vi "Splashscreen.vi"(1 "Mode":enum16{"splash", "dialog"}(ring)) -> ()   [LabVIEW 2009]
panel:
  in  "OK Button":bool
  # "PCI"
  # "Physikalisch-Chemisches Institut\nUniversität Heidelberg\nIm Neuenheimer Feld 253"
  # "This software has been developed as tool for optical single molecule spectroscopy within\nthe group of Prof. Dr. J. Wolfrum and Prof. Dr. M. Sauer. It contains all state of the art\ndata acqusition and analysis algorythms developed and used by our workgroup for our \nsingle molecule studies.\n\nThe people mainly involved in these developments through\ndiscussion, experiments and software development are:\n\nDirk-Peter Herten, Philip Tinnefeld, Kenneth D. Weston, Christian Müller,\nChristian Roth, Oliver Piestert and Markus Sauer\n\nPicoQuant HydraHarp modifications by Christian Steinhauer\n\nCopyright (c) 1999, 2000, 2001, 2002, 2003 Physikalisch-Chemisches Institut\nAll rights reserved."
  # "NO WARRANITIES. NOT FOR RESALE.\nCOPIES AND DISTRIBUTION OF THIS SOFTWARE\nIS ONLY ALLOWED WITH EXPLICIT\nPERMITION BY ONE OF ABOVE LISTED PERSONS."
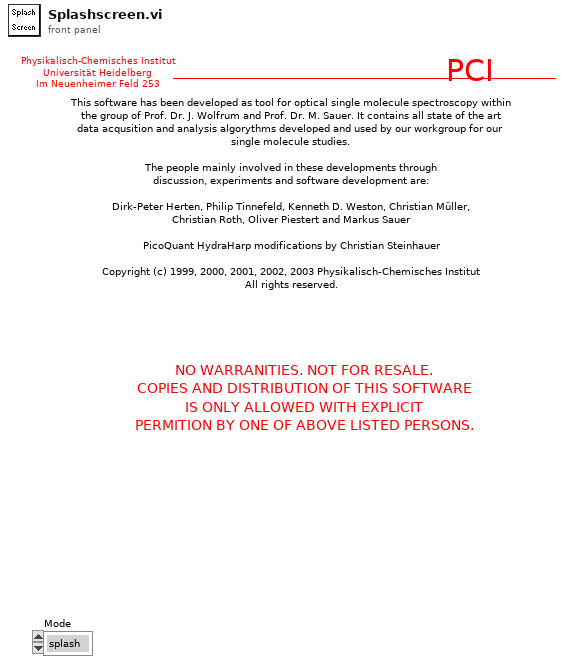
[diagram p1: front panel]
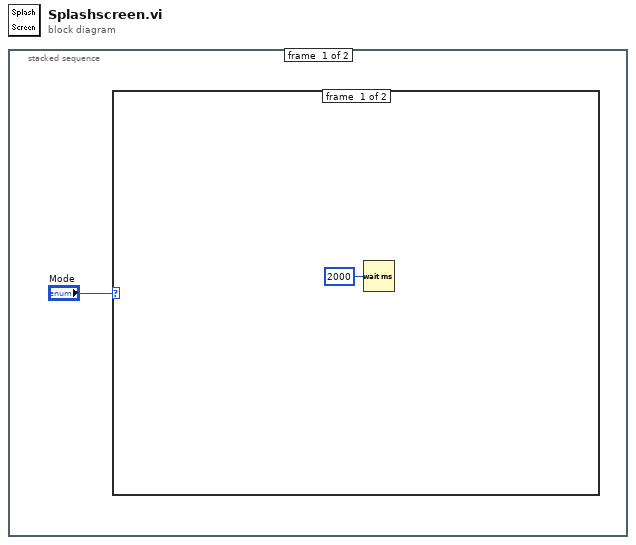
[diagram p0: block diagram]
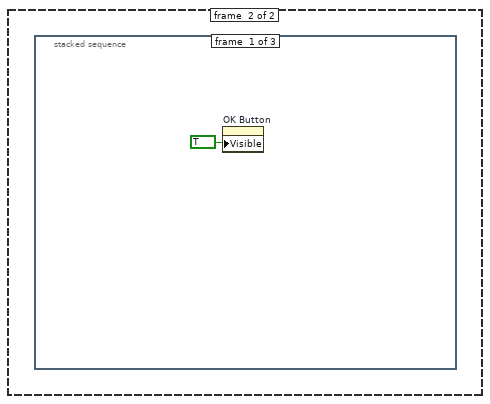
[diagram p2: hidden frame]
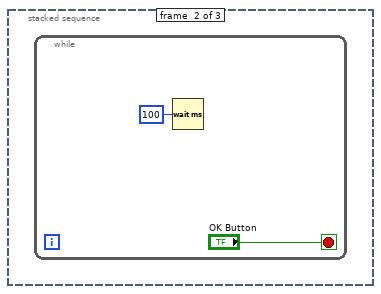
[diagram p3: hidden frame]
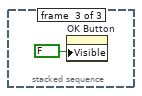
[diagram p4: hidden frame]
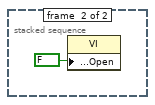
[diagram p5: hidden frame]
diagram:
  n1 = stacked-sequence {
    frame #0 {
      n2 = case shown="\"dialog\"" "Mode" {
        frame #0 {
          n3 = Wait (ms)(milliseconds to wait=u32 2000) -> ()  [unwired: 1 out]
        }
        frame #1 {
          n4 = stacked-sequence {
            frame #0 {
              n5 = property on="OK Button" class="Boolean"("Visible"=TRUE) -> ()  [unwired: 2 in, 2 out]
            }
            frame #1 {
              n6 = while {
                stop <- "OK Button" stop-if-true
                n7 = Wait (ms)(milliseconds to wait=u32 100) -> ()  [unwired: 1 out]
              }
            }
            frame #2 {
              n8 = property on="OK Button" class="Boolean"("Visible"=FALSE) -> ()  [unwired: 2 in, 2 out]
            }
          }
        }
      }
    }
    frame #1 {
      n9 = property class="VI"("Front Panel Window:Open"=FALSE) -> ()  [unwired: 2 in, 2 out]
    }
  }
